vi "ProcessDefaultQueueName.vi"() -> (0 "processDefaultQueueName":string)   [LabVIEW 2026, in "Lumberjack.lvlib"]
doc: "Returns the fixed process-global named-queue key for the default Logger store. Shared by SetProcessDefault, GetProcessDefault, and ClearProcessDefault so all three address the same single-element queue."
uses:
  Lumberjack.lvlib
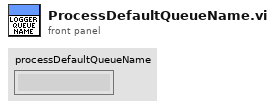
[diagram p1: front panel]
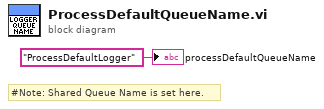
[diagram p0: block diagram]
diagram:
  # "#Note: Shared Queue Name is set here."
  "processDefaultQueueName" <- "ProcessDefaultLogger" ("processDefaultQueueName")
